vi "Autonomous State Machine .vi"   [LabVIEW 2014]
doc: "This VI is called when autonomous begins, and will automatically be terminated when autonomous ends. You can carry out timed or sensor driven robot movement independently without needing to return to the caller."
uses:
  <vilib>/Rock Robotics/WPI/RobotDrive/WPI_RobotDriveGetSetRefNum.vi
  Robot Global Data.vi
panel:
  # "Be sure to right-click and choose Data Operations>>Make Current Value default if you want to save the array values with the VI"
types:
  T1 = typedef "WPI_MotorControlDeviceRef.ctl" = cluster{"DeviceStatus":errorcluster, "Type":T2, "PWM":cluster{"Controller":T3, "PWM Channel":T4, "DeadBand":T5}, "CAN":cluster{"Device Number":u8, "Control Mode":T6, "Semaphore":T7, "Max Vout":dbl, "TalonSRX Control Mode":T8}, "Invert":bool, "TransformRef":T9, "InvTransformRef":T9}
  T2 = typedef "WPI_MotorControlType.ctl" = enum16{"PWM", "CAN", "CANTalonSRX"}
  T3 = typedef "FPGA_TypedefDigitalModule.ctl" = enum16{"Controller 1"}
  T4 = typedef "FPGA_DIOPWMChannel.ctl" = enum8{"PWM 0", "PWM 1", "PWM 2", "PWM 3", "PWM 4", "PWM 5", "PWM 6", "PWM 7", "PWM 8", "PWM 9", "PWM MXP 0", "PWM MXP 1", "PWM MXP 2", "PWM MXP 3", "PWM MXP 4", "PWM MXP 5", "PWM MXP 6", "PWM MXP 7", "PWM MXP 8", "PWM MXP 9", "Invalid"}
  T5 = typedef "WPI_PWMDeadband.ctl" = cluster{"Name":string, "maxPositivePwm":i32, "minPositivePwm":i32, "centerPwm":i32, "maxNegativePwm":i32, "minNegativePwm":i32, "angularRange":u16}
  T6 = typedef "WPI_CANJaguar_ControlMode.ctl" = enum8{"Percent VBus", "Current", "Speed", "Position", "Voltage"}
  T7 = typedef "Semaphore RefNum" = refnum<k1>
  T8 = typedef "WPI_CANTalonSRX_APIControlMode.ctl" = enum8{"Percent VBus", "Speed", "Position", "Slave", "Unchanged / Invalid"}
  T9 = typedef "WPI_PWMTransform_ConPane.ctl" = refnum<vi>
  T10 = typedef "WPI_RobotDriveDevRef.ctl" = cluster{"DevStatus":errorcluster, "Motors[]":T1[], "Square Inputs":bool, "Max Output":dbl}
  T11 = typedef "WPI_DigitalInputDevRef.ctl" = cluster{"DevStatus":errorcluster, "DIO Channel":T12, "Controller":T3}
  T12 = typedef "FPGA_DIOChannel.ctl" = enum8{"DIO 0", "DIO 1", "DIO 2", "DIO 3", "DIO 4", "DIO 5", "DIO 6", "DIO 7", "DIO 8", "DIO 9", "DIO MXP 0", "DIO MXP 1", "DIO MXP 2", "DIO MXP 3", "DIO MXP 4", "DIO MXP 5", "DIO MXP 6", "DIO MXP 7", "DIO MXP 8", "DIO MXP 9", "DIO MXP 10", "DIO MXP 11", "DIO MXP 12", "DIO MXP 13", "DIO MXP 14", "DIO MXP 15", "Invalid"}
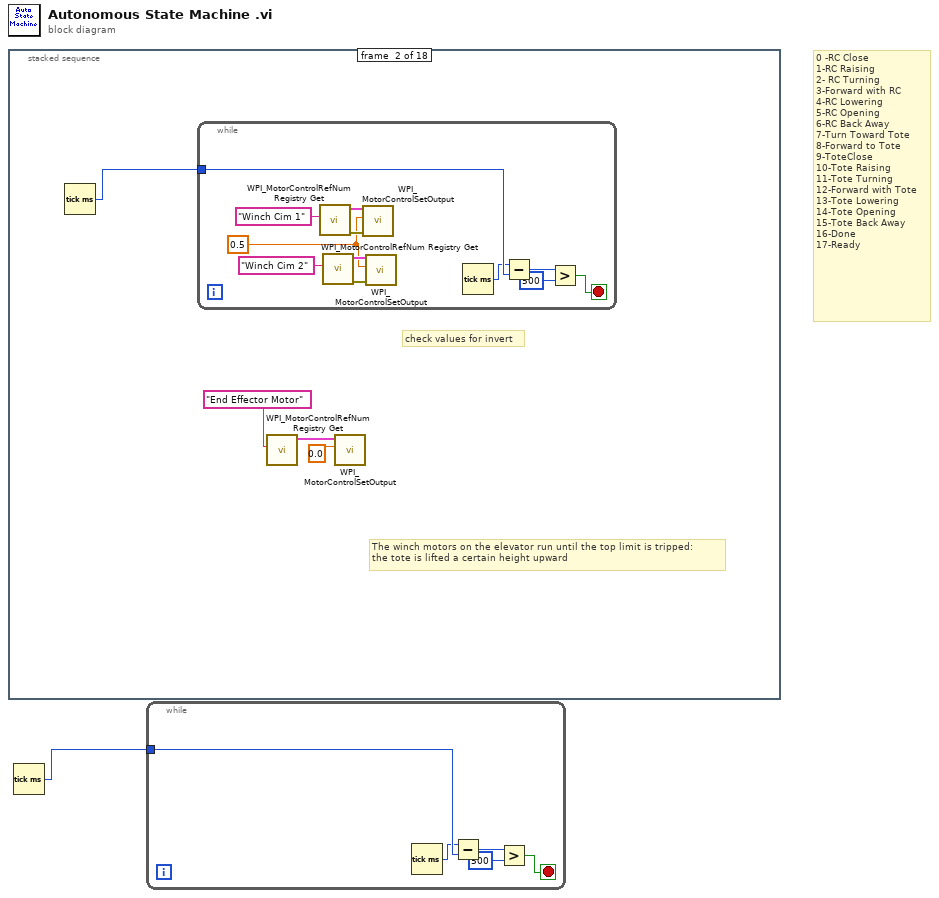
[diagram p0: block diagram]
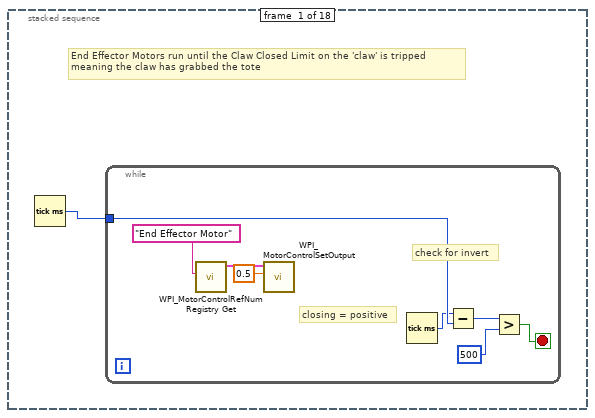
[diagram p2: hidden frame]
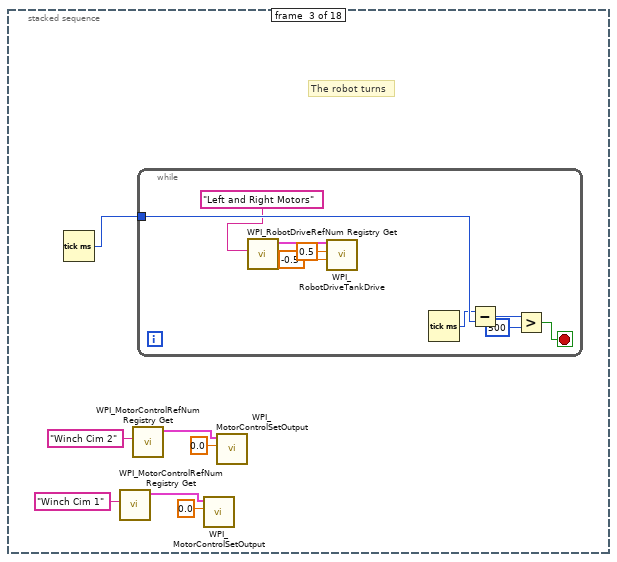
[diagram p3: hidden frame]
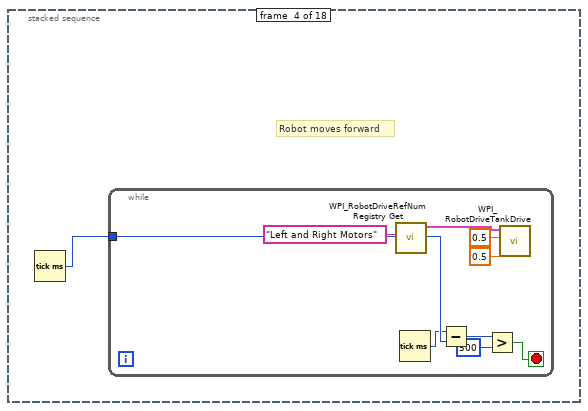
[diagram p4: hidden frame]
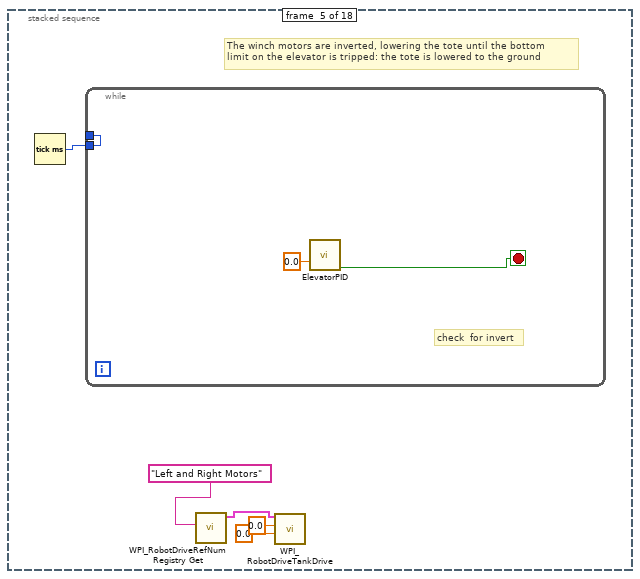
[diagram p5: hidden frame]
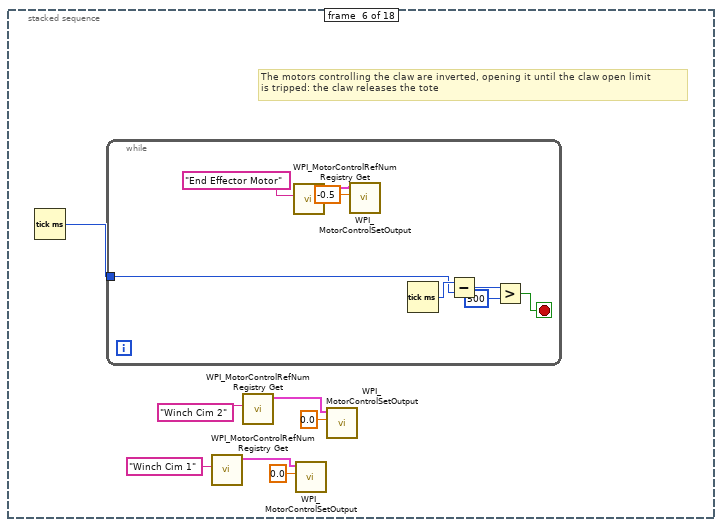
[diagram p6: hidden frame]
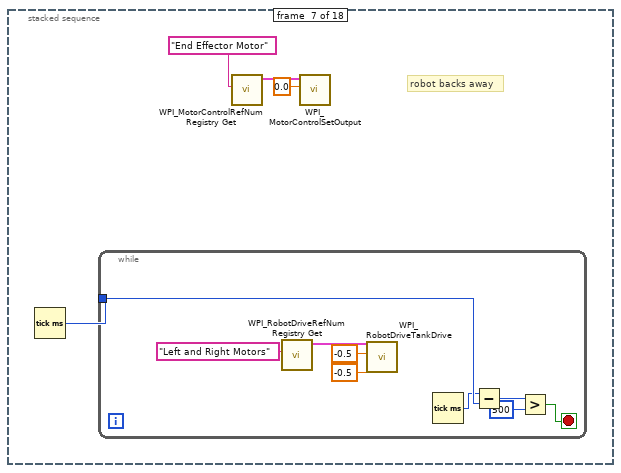
[diagram p7: hidden frame]
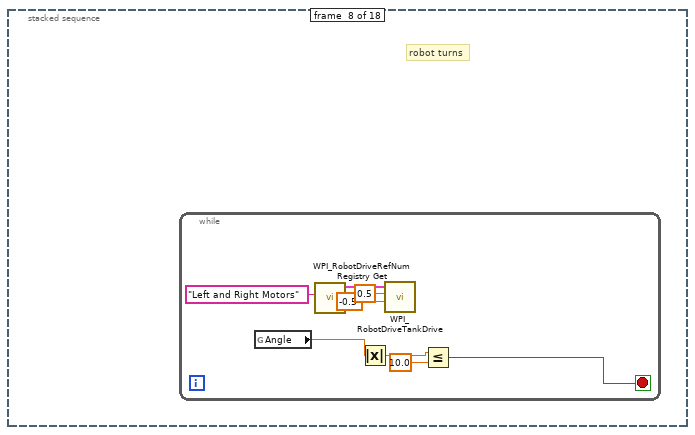
[diagram p8: hidden frame]
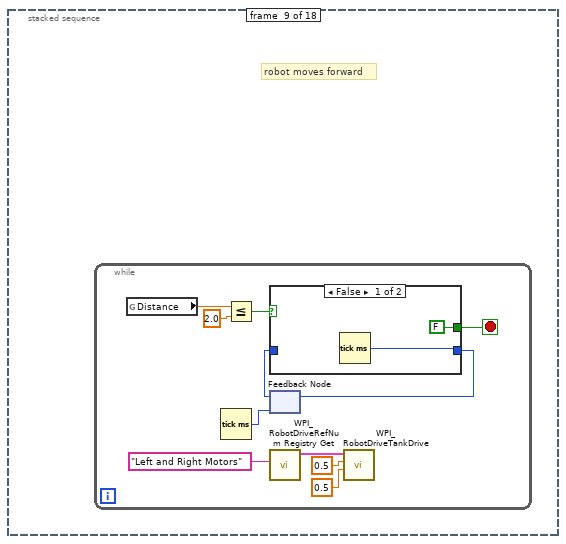
[diagram p9: hidden frame]
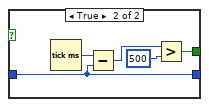
[diagram p10: hidden frame]
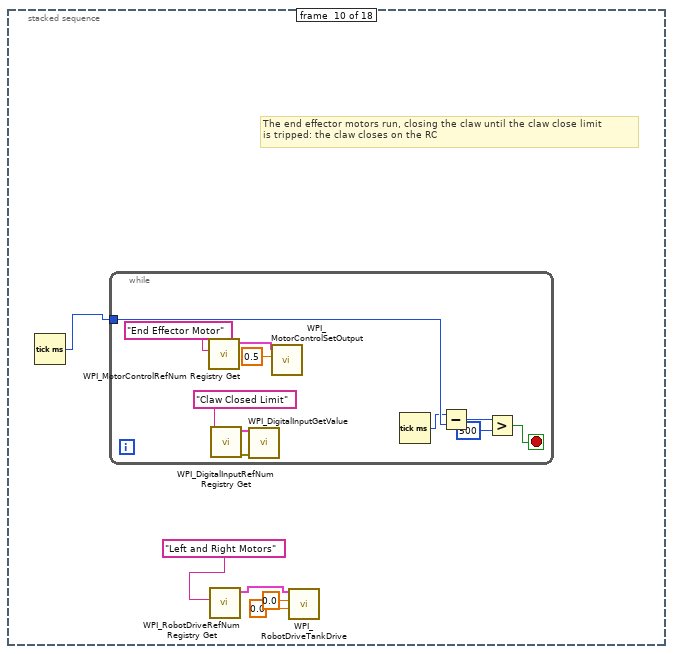
[diagram p11: hidden frame]
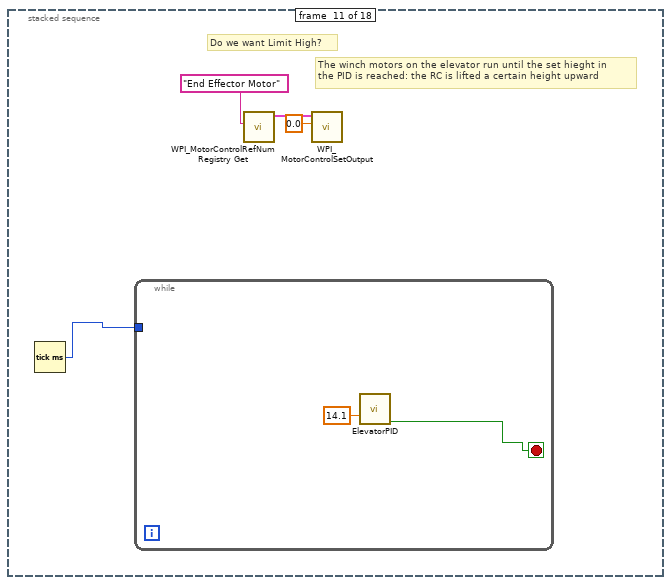
[diagram p12: hidden frame]
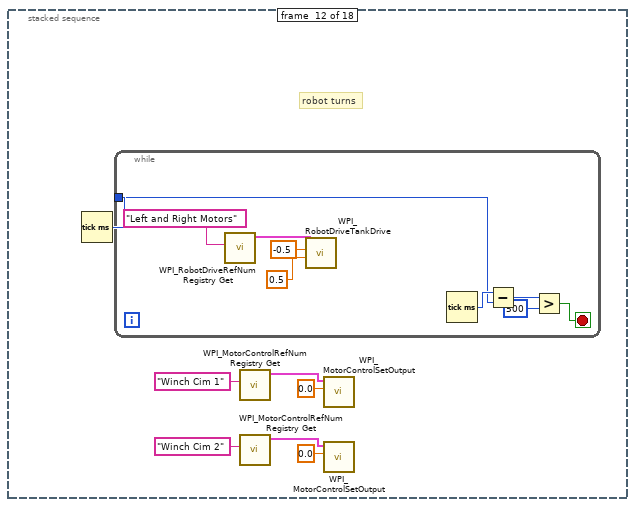
[diagram p13: hidden frame]
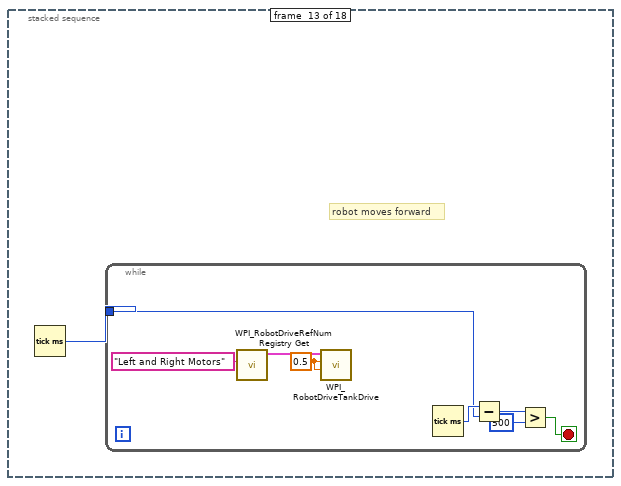
[diagram p14: hidden frame]
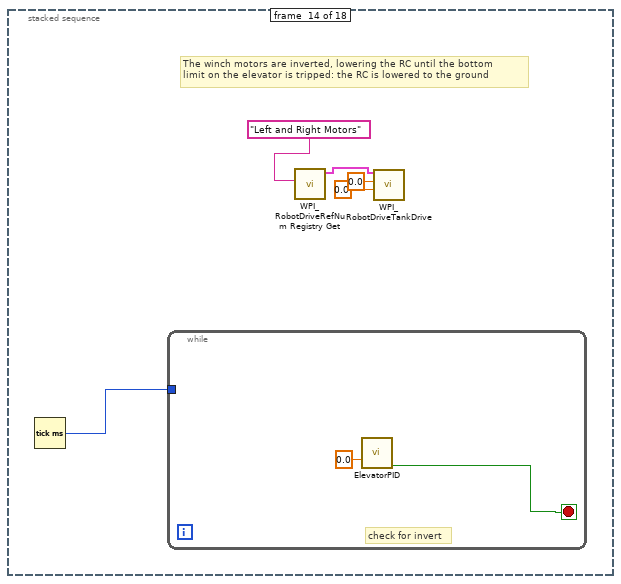
[diagram p15: hidden frame]
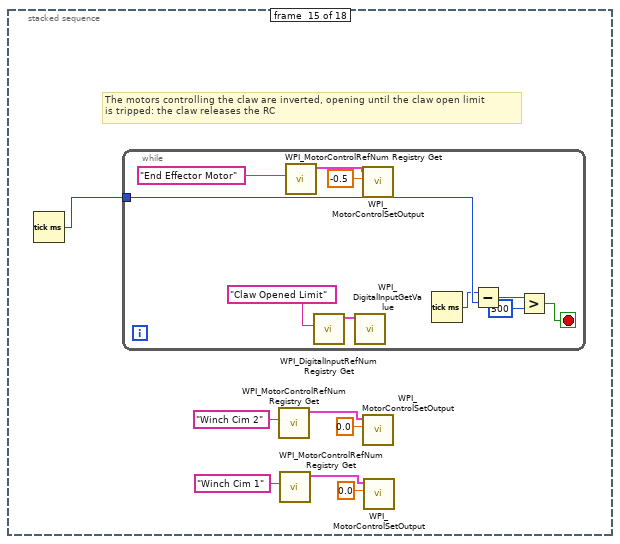
[diagram p16: hidden frame]
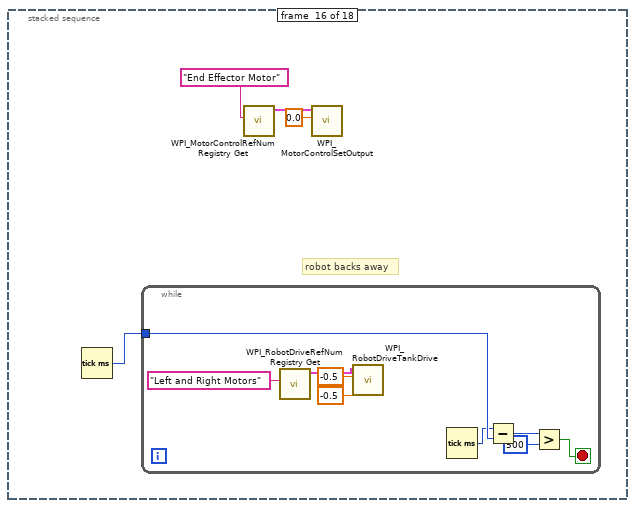
[diagram p17: hidden frame]
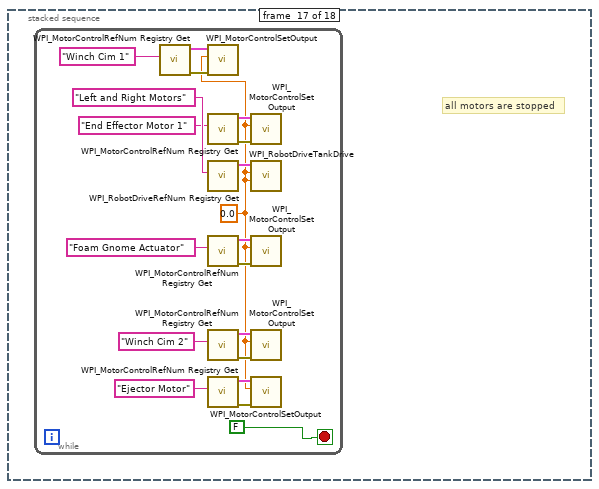
[diagram p18: hidden frame]
diagram:
  # "0 -RC Close\n1-RC Raising\n2- RC Turning\n3-Forward with RC\n4-RC Lowering\n5-RC Opening\n6-RC Back Away\n7-Turn Toward Tote\n8-Forward to Tote\n9-ToteClose\n10-Tote Raising\n11-Tote Turning\n12-Forward with Tote\n13-Tote Lowering\n14-Tote Opening\n15-Tote Back Away\n16-Done\n17-Ready"
  n1 = stacked-sequence {
    frame #0 {
      # "End Effector Motors run until the Claw Closed Limit on the 'claw' is tripped\nmeaning the claw has grabbed the tote"
      n2 = Tick Count (ms)() -> (millisecond timer value=w2:u32)
      n3 = while {
        tunnel: w2 -> [w7]
        stop <- w8 stop-if-true
        # "closing = positive"
        # "check for invert"
        n4 = call <vilib>:"WPI_MotorControlRefNum Registry Get.vi"("refnum name"="End Effector Motor") -> ("MotorControlDevRef"=w3:T1)  [unwired: 9 in, 1 out]
        n5 = call <vilib>:"WPI_MotorControlSetOutput.vi"("Output"=0.5, "MotorControlDevRef"=w3) -> ()  [unwired: 7 in, 3 out]
        n6 = Tick Count (ms)() -> (millisecond timer value=w6:u32)
        n7 = Subtract(x=w6, y=w7) -> (x-y=w10:u32)
        n8 = Greater?(x=w10, y=u32 500) -> (0:w8:bool)
      }
    }
    frame #1 {
      # "The winch motors on the elevator run until the top limit is tripped: \nthe tote is lifted a certain height upward"
      # "check values for invert"
      n9 = Tick Count (ms)() -> (millisecond timer value=w11:u32)
      n10 = while {
        tunnel: w11 -> [w23]
        stop <- w24 stop-if-true
        w15 = 0.5
        n11 = call <vilib>:"WPI_MotorControlRefNum Registry Get.vi"("refnum name"="Winch Cim 1") -> ("error out"=w20:errorcluster, "MotorControlDevRef"=w19:T1)  [unwired: 9 in]
        n12 = call <vilib>:"WPI_MotorControlRefNum Registry Get.vi"("refnum name"="Winch Cim 2") -> ("error out"=w17:errorcluster, "MotorControlDevRef"=w16:T1)  [unwired: 9 in]
        n13 = call <vilib>:"WPI_MotorControlSetOutput.vi"("error in (no error)"=w20, "Output"=w15, "MotorControlDevRef"=w19) -> ()  [unwired: 6 in, 3 out]
        n14 = call <vilib>:"WPI_MotorControlSetOutput.vi"("error in (no error)"=w17, "Output"=w15, "MotorControlDevRef"=w16) -> ()  [unwired: 6 in, 3 out]
        n15 = Tick Count (ms)() -> (millisecond timer value=w22:u32)
        n16 = Subtract(x=w22, y=w23) -> (x-y=w26:u32)
        n17 = Greater?(x=w26, y=u32 500) -> (0:w24:bool)
      }
      n18 = call <vilib>:"WPI_MotorControlRefNum Registry Get.vi"("refnum name"="End Effector Motor") -> ("MotorControlDevRef"=w12:T1)  [unwired: 9 in, 1 out]
      n19 = call <vilib>:"WPI_MotorControlSetOutput.vi"("Output"=0.0, "MotorControlDevRef"=w12) -> ()  [unwired: 7 in, 3 out]
    }
    frame #2 {
      # "The robot turns"
      n20 = Tick Count (ms)() -> (millisecond timer value=w33:u32)
      n21 = call <vilib>:"WPI_MotorControlRefNum Registry Get.vi"("refnum name"="Winch Cim 1") -> ("MotorControlDevRef"=w28:T1)  [unwired: 9 in, 1 out]
      n22 = call <vilib>:"WPI_MotorControlRefNum Registry Get.vi"("refnum name"="Winch Cim 2") -> ("MotorControlDevRef"=w31:T1)  [unwired: 9 in, 1 out]
      n23 = while {
        tunnel: w33 -> [w39]
        stop <- w40 stop-if-true
        n24 = call <vilib>:"WPI_RobotDriveRefNum Registry Get.vi"("refnum name"="Left and Right Motors") -> ("RobotDriveDevRef"=w37:T10)  [unwired: 9 in, 1 out]
        n25 = call <vilib>:"WPI_RobotDriveTankDrive.vi"("Right axis value"=-0.5, "Left axis value"=0.5, "RobotDriveDevRef"=w37) -> ()  [unwired: 6 in, 3 out]
        n26 = Tick Count (ms)() -> (millisecond timer value=w38:u32)
        n27 = Subtract(x=w38, y=w39) -> (x-y=w42:u32)
        n28 = Greater?(x=w42, y=u32 500) -> (0:w40:bool)
      }
      n29 = call <vilib>:"WPI_MotorControlSetOutput.vi"("Output"=0.0, "MotorControlDevRef"=w28) -> ()  [unwired: 7 in, 3 out]
      n30 = call <vilib>:"WPI_MotorControlSetOutput.vi"("Output"=0.0, "MotorControlDevRef"=w31) -> ()  [unwired: 7 in, 3 out]
    }
    frame #3 {
      # "Robot moves forward"
      n31 = Tick Count (ms)() -> (millisecond timer value=w43:u32)
      n32 = while {
        tunnel: w43 -> [w49]
        stop <- w50 stop-if-true
        n33 = call <vilib>:"WPI_RobotDriveRefNum Registry Get.vi"("refnum name"="Left and Right Motors") -> ("RobotDriveDevRef"=w47:T10)  [unwired: 9 in, 1 out]
        n34 = Tick Count (ms)() -> (millisecond timer value=w48:u32)
        n35 = Subtract(x=w48, y=w49) -> (x-y=w52:u32)
        n36 = Greater?(x=w52, y=u32 500) -> (0:w50:bool)
        n37 = call <vilib>:"WPI_RobotDriveTankDrive.vi"("Right axis value"=0.5, "Left axis value"=0.5, "RobotDriveDevRef"=w47) -> ()  [unwired: 6 in, 3 out]
      }
    }
    frame #4 {
      # "The winch motors are inverted, lowering the tote until the bottom \nlimit on the elevator is tripped: the tote is lowered to the ground"
      n38 = Tick Count (ms)() -> (millisecond timer value=w57:u32)
      n39 = while {
        tunnel: [w60] -> _
        tunnel: w57 -> [w60]
        stop <- w58 stop-if-true
        # "check  for invert"
        n40 = call "ElevatorPID.vi"("Elevator Setpoint"=0.0) -> ("At Setpoint"=w58:bool)  [unwired: 14 in]
      }
      n41 = call <vilib>:"WPI_RobotDriveRefNum Registry Get.vi"("refnum name"="Left and Right Motors") -> ("RobotDriveDevRef"=w56:T10)  [unwired: 9 in, 1 out]
      n42 = call <vilib>:"WPI_RobotDriveTankDrive.vi"("Right axis value"=0.0, "Left axis value"=0.0, "RobotDriveDevRef"=w56) -> ()  [unwired: 6 in, 3 out]
    }
    frame #5 {
      # "The motors controlling the claw are inverted, opening it until the claw open limit\nis tripped: the claw releases the tote"
      n43 = Tick Count (ms)() -> (millisecond timer value=w67:u32)
      n44 = while {
        tunnel: w67 -> [w68]
        stop <- w73 stop-if-true
        n45 = call <vilib>:"WPI_MotorControlRefNum Registry Get.vi"("refnum name"="End Effector Motor") -> ("MotorControlDevRef"=w70:T1)  [unwired: 9 in, 1 out]
        n46 = call <vilib>:"WPI_MotorControlSetOutput.vi"("Output"=-0.5, "MotorControlDevRef"=w70) -> ()  [unwired: 7 in, 3 out]
        n47 = Tick Count (ms)() -> (millisecond timer value=w72:u32)
        n48 = Subtract(x=w72, y=w68) -> (x-y=w75:u32)
        n49 = Greater?(x=w75, y=u32 500) -> (0:w73:bool)
      }
      n50 = call <vilib>:"WPI_MotorControlRefNum Registry Get.vi"("refnum name"="Winch Cim 1") -> ("MotorControlDevRef"=w62:T1)  [unwired: 9 in, 1 out]
      n51 = call <vilib>:"WPI_MotorControlRefNum Registry Get.vi"("refnum name"="Winch Cim 2") -> ("MotorControlDevRef"=w65:T1)  [unwired: 9 in, 1 out]
      n52 = call <vilib>:"WPI_MotorControlSetOutput.vi"("Output"=0.0, "MotorControlDevRef"=w62) -> ()  [unwired: 7 in, 3 out]
      n53 = call <vilib>:"WPI_MotorControlSetOutput.vi"("Output"=0.0, "MotorControlDevRef"=w65) -> ()  [unwired: 7 in, 3 out]
    }
    frame #6 {
      # "robot backs away"
      n54 = Tick Count (ms)() -> (millisecond timer value=w79:u32)
      n55 = while {
        tunnel: w79 -> [w85]
        stop <- w86 stop-if-true
        n56 = call <vilib>:"WPI_RobotDriveRefNum Registry Get.vi"("refnum name"="Left and Right Motors") -> ("RobotDriveDevRef"=w83:T10)  [unwired: 9 in, 1 out]
        n57 = call <vilib>:"WPI_RobotDriveTankDrive.vi"("Right axis value"=-0.5, "Left axis value"=-0.5, "RobotDriveDevRef"=w83) -> ()  [unwired: 6 in, 3 out]
        n58 = Tick Count (ms)() -> (millisecond timer value=w84:u32)
        n59 = Subtract(x=w84, y=w85) -> (x-y=w88:u32)
        n60 = Greater?(x=w88, y=u32 500) -> (0:w86:bool)
      }
      n61 = call <vilib>:"WPI_MotorControlRefNum Registry Get.vi"("refnum name"="End Effector Motor") -> ("MotorControlDevRef"=w76:T1)  [unwired: 9 in, 1 out]
      n62 = call <vilib>:"WPI_MotorControlSetOutput.vi"("Output"=0.0, "MotorControlDevRef"=w76) -> ()  [unwired: 7 in, 3 out]
    }
    frame #7 {
      # "robot turns"
      n63 = while {
        stop <- w89 stop-if-true
        n64 = global read "Robot Global Data.vi" "Angle"() -> (w90:dbl)
        n65 = call <vilib>:"WPI_RobotDriveRefNum Registry Get.vi"("refnum name"="Left and Right Motors") -> ("RobotDriveDevRef"=w96:T10)  [unwired: 9 in, 1 out]
        n66 = Absolute Value(x=w90) -> (abs(x)=w91:dbl)
        n67 = call <vilib>:"WPI_RobotDriveTankDrive.vi"("Right axis value"=-0.5, "Left axis value"=0.5, "RobotDriveDevRef"=w96) -> ()  [unwired: 6 in, 3 out]
        n68 = Less Or Equal?(x=w91, y=10.0) -> (x <= y?=w89:bool)
      }
    }
    frame #8 {
      # "robot moves forward"
      n69 = while {
        stop <- w100 stop-if-true
        n70 = global read "Robot Global Data.vi" "Distance"() -> (w103:dbl)
        n71 = Tick Count (ms)() -> (millisecond timer value=w97:u32)
        n72 = Less Or Equal?(x=w103, y=2.0) -> (x <= y?=w101:bool)
        n73 = feedback #1(w97) -> (w98:u32)
        n74 = case shown="False" w101 {
          tunnel: [w108 w110] -> w99
          tunnel: [FALSE w111] -> w100
          tunnel: w98 -> [_ w110]
          frame False {
            n75 = Tick Count (ms)() -> (millisecond timer value=w108:u32)
          }
          frame True {
            n76 = Tick Count (ms)() -> (millisecond timer value=w112:u32)
            n77 = Subtract(x=w112, y=w110) -> (x-y=w114:u32)
            n78 = Greater?(x=w114, y=u32 500) -> (0:w111:bool)
          }
        }
        n79 = feedback-in #1(w99) -> ()
        n80 = call <vilib>:"WPI_RobotDriveRefNum Registry Get.vi"("refnum name"="Left and Right Motors") -> ("RobotDriveDevRef"=w107:T10)  [unwired: 9 in, 1 out]
        n81 = call <vilib>:"WPI_RobotDriveTankDrive.vi"("Right axis value"=0.5, "Left axis value"=0.5, "RobotDriveDevRef"=w107) -> ()  [unwired: 6 in, 3 out]
      }
    }
    frame #9 {
      # "The end effector motors run, closing the claw until the claw close limit \nis tripped: the claw closes on the RC"
      n82 = Tick Count (ms)() -> (millisecond timer value=w119:u32)
      n83 = while {
        tunnel: w119 -> [w127]
        stop <- w128 stop-if-true
        n84 = call <vilib>:"WPI_MotorControlRefNum Registry Get.vi"("refnum name"="End Effector Motor") -> ("MotorControlDevRef"=w123:T1)  [unwired: 9 in, 1 out]
        n85 = call <vilib>:"WPI_DigitalInputRefNum Registry Get.vi"("refnum name"="Claw Closed Limit") -> ("error out"=w121:errorcluster, "DigitalInputDevRef"=w122:T11)  [unwired: 9 in]
        n86 = call <vilib>:"WPI_DigitalInputGetValue.vi"("error in (no error)"=w121, "DigitalInputDevRef"=w122) -> ()  [unwired: 7 in, 3 out]
        n87 = call <vilib>:"WPI_MotorControlSetOutput.vi"("Output"=0.5, "MotorControlDevRef"=w123) -> ()  [unwired: 7 in, 3 out]
        n88 = Tick Count (ms)() -> (millisecond timer value=w126:u32)
        n89 = Subtract(x=w126, y=w127) -> (x-y=w130:u32)
        n90 = Greater?(x=w130, y=u32 500) -> (0:w128:bool)
      }
      n91 = call <vilib>:"WPI_RobotDriveRefNum Registry Get.vi"("refnum name"="Left and Right Motors") -> ("RobotDriveDevRef"=w118:T10)  [unwired: 9 in, 1 out]
      n92 = call <vilib>:"WPI_RobotDriveTankDrive.vi"("Right axis value"=0.0, "Left axis value"=0.0, "RobotDriveDevRef"=w118) -> ()  [unwired: 6 in, 3 out]
    }
    frame #10 {
      # "The winch motors on the elevator run until the set hieght in \nthe PID is reached: the RC is lifted a certain height upward"
      # "Do we want Limit High?"
      n93 = Tick Count (ms)() -> (millisecond timer value=w134:u32)
      n94 = while {
        tunnel: w134 -> [_]
        stop <- w135 stop-if-true
        n95 = call "ElevatorPID.vi"("Elevator Setpoint"=14.1) -> ("At Setpoint"=w135:bool)  [unwired: 14 in]
      }
      n96 = call <vilib>:"WPI_MotorControlRefNum Registry Get.vi"("refnum name"="End Effector Motor") -> ("MotorControlDevRef"=w133:T1)  [unwired: 9 in, 1 out]
      n97 = call <vilib>:"WPI_MotorControlSetOutput.vi"("Output"=0.0, "MotorControlDevRef"=w133) -> ()  [unwired: 7 in, 3 out]
    }
    frame #11 {
      # "robot turns"
      n98 = Tick Count (ms)() -> (millisecond timer value=w143:u32)
      n99 = while {
        tunnel: w143 -> [w148]
        stop <- w150 stop-if-true
        n100 = call <vilib>:"WPI_RobotDriveRefNum Registry Get.vi"("refnum name"="Left and Right Motors") -> ("RobotDriveDevRef"=w147:T10)  [unwired: 9 in, 1 out]
        n101 = call <vilib>:"WPI_RobotDriveTankDrive.vi"("Right axis value"=0.5, "Left axis value"=-0.5, "RobotDriveDevRef"=w147) -> ()  [unwired: 6 in, 3 out]
        n102 = Tick Count (ms)() -> (millisecond timer value=w149:u32)
        n103 = Subtract(x=w149, y=w148) -> (x-y=w152:u32)
        n104 = Greater?(x=w152, y=u32 500) -> (0:w150:bool)
      }
      n105 = call <vilib>:"WPI_MotorControlRefNum Registry Get.vi"("refnum name"="Winch Cim 1") -> ("MotorControlDevRef"=w141:T1)  [unwired: 9 in, 1 out]
      n106 = call <vilib>:"WPI_MotorControlRefNum Registry Get.vi"("refnum name"="Winch Cim 2") -> ("MotorControlDevRef"=w138:T1)  [unwired: 9 in, 1 out]
      n107 = call <vilib>:"WPI_MotorControlSetOutput.vi"("Output"=0.0, "MotorControlDevRef"=w141) -> ()  [unwired: 7 in, 3 out]
      n108 = call <vilib>:"WPI_MotorControlSetOutput.vi"("Output"=0.0, "MotorControlDevRef"=w138) -> ()  [unwired: 7 in, 3 out]
    }
    frame #12 {
      # "robot moves forward"
      n109 = Tick Count (ms)() -> (millisecond timer value=w153:u32)
      n110 = while {
        tunnel: w153 -> [w157]
        stop <- w159 stop-if-true
        w154 = 0.5 ("Left axis value")
        n111 = call <vilib>:"WPI_RobotDriveRefNum Registry Get.vi"("refnum name"="Left and Right Motors") -> ("RobotDriveDevRef"=w156:T10)  [unwired: 9 in, 1 out]
        n112 = call <vilib>:"WPI_RobotDriveTankDrive.vi"("Right axis value"=w154, "Left axis value"=w154, "RobotDriveDevRef"=w156) -> ()  [unwired: 6 in, 3 out]
        n113 = Tick Count (ms)() -> (millisecond timer value=w158:u32)
        n114 = Subtract(x=w158, y=w157) -> (x-y=w161:u32)
        n115 = Greater?(x=w161, y=u32 500) -> (0:w159:bool)
      }
    }
    frame #13 {
      # "The winch motors are inverted, lowering the RC until the bottom \nlimit on the elevator is tripped: the RC is lowered to the ground"
      n116 = Tick Count (ms)() -> (millisecond timer value=w166:u32)
      n117 = while {
        tunnel: w166 -> [_]
        stop <- w167 stop-if-true
        # "check for invert"
        n118 = call "ElevatorPID.vi"("Elevator Setpoint"=0.0) -> ("At Setpoint"=w167:bool)  [unwired: 14 in]
      }
      n119 = call <vilib>:"WPI_RobotDriveRefNum Registry Get.vi"("refnum name"="Left and Right Motors") -> ("RobotDriveDevRef"=w165:T10)  [unwired: 9 in, 1 out]
      n120 = call <vilib>:"WPI_RobotDriveTankDrive.vi"("Right axis value"=0.0, "Left axis value"=0.0, "RobotDriveDevRef"=w165) -> ()  [unwired: 6 in, 3 out]
    }
    frame #14 {
      # "The motors controlling the claw are inverted, opening until the claw open limit\nis tripped: the claw releases the RC"
      n121 = Tick Count (ms)() -> (millisecond timer value=w175:u32)
      n122 = while {
        tunnel: w175 -> [w182]
        stop <- w183 stop-if-true
        n123 = call <vilib>:"WPI_MotorControlRefNum Registry Get.vi"("refnum name"="End Effector Motor") -> ("MotorControlDevRef"=w176:T1)  [unwired: 9 in, 1 out]
        n124 = call <vilib>:"WPI_DigitalInputRefNum Registry Get.vi"("refnum name"="Claw Opened Limit") -> ("DigitalInputDevRef"=w179:T11)  [unwired: 9 in, 1 out]
        n125 = call <vilib>:"WPI_DigitalInputGetValue.vi"("DigitalInputDevRef"=w179) -> ()  [unwired: 8 in, 3 out]
        n126 = call <vilib>:"WPI_MotorControlSetOutput.vi"("Output"=-0.5, "MotorControlDevRef"=w176) -> ()  [unwired: 7 in, 3 out]
        n127 = Tick Count (ms)() -> (millisecond timer value=w181:u32)
        n128 = Subtract(x=w181, y=w182) -> (x-y=w185:u32)
        n129 = Greater?(x=w185, y=u32 500) -> (0:w183:bool)
      }
      n130 = call <vilib>:"WPI_MotorControlRefNum Registry Get.vi"("refnum name"="Winch Cim 2") -> ("MotorControlDevRef"=w173:T1)  [unwired: 9 in, 1 out]
      n131 = call <vilib>:"WPI_MotorControlRefNum Registry Get.vi"("refnum name"="Winch Cim 1") -> ("MotorControlDevRef"=w170:T1)  [unwired: 9 in, 1 out]
      n132 = call <vilib>:"WPI_MotorControlSetOutput.vi"("Output"=0.0, "MotorControlDevRef"=w173) -> ()  [unwired: 7 in, 3 out]
      n133 = call <vilib>:"WPI_MotorControlSetOutput.vi"("Output"=0.0, "MotorControlDevRef"=w170) -> ()  [unwired: 7 in, 3 out]
    }
    frame #15 {
      # "robot backs away"
      n134 = Tick Count (ms)() -> (millisecond timer value=w189:u32)
      n135 = while {
        tunnel: w189 -> [w195]
        stop <- w196 stop-if-true
        n136 = call <vilib>:"WPI_RobotDriveRefNum Registry Get.vi"("refnum name"="Left and Right Motors") -> ("RobotDriveDevRef"=w193:T10)  [unwired: 9 in, 1 out]
        n137 = call <vilib>:"WPI_RobotDriveTankDrive.vi"("Right axis value"=-0.5, "Left axis value"=-0.5, "RobotDriveDevRef"=w193) -> ()  [unwired: 6 in, 3 out]
        n138 = Tick Count (ms)() -> (millisecond timer value=w194:u32)
        n139 = Subtract(x=w194, y=w195) -> (x-y=w198:u32)
        n140 = Greater?(x=w198, y=u32 500) -> (0:w196:bool)
      }
      n141 = call <vilib>:"WPI_MotorControlRefNum Registry Get.vi"("refnum name"="End Effector Motor") -> ("MotorControlDevRef"=w186:T1)  [unwired: 9 in, 1 out]
      n142 = call <vilib>:"WPI_MotorControlSetOutput.vi"("Output"=0.0, "MotorControlDevRef"=w186) -> ()  [unwired: 7 in, 3 out]
    }
    frame #16 {
      # "all motors are stopped"
      n143 = while {
        stop <- FALSE stop-if-true
        w199 = 0.0
        n144 = call <vilib>:"WPI_MotorControlRefNum Registry Get.vi"("refnum name"="Winch Cim 1") -> ("error out"=w208:errorcluster, "MotorControlDevRef"=w207:T1)  [unwired: 9 in]
        n145 = call <vilib>:"WPI_MotorControlSetOutput.vi"("error in (no error)"=w208, "Output"=w199, "MotorControlDevRef"=w207) -> ()  [unwired: 6 in, 3 out]
        n146 = call <vilib>:"WPI_MotorControlRefNum Registry Get.vi"("refnum name"="End Effector Motor 1") -> ("error out"=w214:errorcluster, "MotorControlDevRef"=w213:T1)  [unwired: 9 in]
        n147 = call <vilib>:"WPI_RobotDriveRefNum Registry Get.vi"("refnum name"="Left and Right Motors") -> ("RobotDriveDevRef"=w216:T10)  [unwired: 9 in, 1 out]
        n148 = call <vilib>:"WPI_MotorControlRefNum Registry Get.vi"("refnum name"="Foam Gnome Actuator") -> ("error out"=w212:errorcluster, "MotorControlDevRef"=w211:T1)  [unwired: 9 in]
        n149 = call <vilib>:"WPI_MotorControlRefNum Registry Get.vi"("refnum name"="Winch Cim 2") -> ("error out"=w210:errorcluster, "MotorControlDevRef"=w209:T1)  [unwired: 9 in]
        n150 = call <vilib>:"WPI_MotorControlRefNum Registry Get.vi"("refnum name"="Ejector Motor") -> ("error out"=w204:errorcluster, "MotorControlDevRef"=w203:T1)  [unwired: 9 in]
        n151 = call <vilib>:"WPI_MotorControlSetOutput.vi"("error in (no error)"=w214, "Output"=w199, "MotorControlDevRef"=w213) -> ()  [unwired: 6 in, 3 out]
        n152 = call <vilib>:"WPI_RobotDriveTankDrive.vi"("Right axis value"=w199, "Left axis value"=w199, "RobotDriveDevRef"=w216) -> ()  [unwired: 6 in, 3 out]
        n153 = call <vilib>:"WPI_MotorControlSetOutput.vi"("error in (no error)"=w212, "Output"=w199, "MotorControlDevRef"=w211) -> ()  [unwired: 6 in, 3 out]
        n154 = call <vilib>:"WPI_MotorControlSetOutput.vi"("error in (no error)"=w210, "Output"=w199, "MotorControlDevRef"=w209) -> ()  [unwired: 6 in, 3 out]
        n155 = call <vilib>:"WPI_MotorControlSetOutput.vi"("error in (no error)"=w204, "Output"=w199, "MotorControlDevRef"=w203) -> ()  [unwired: 6 in, 3 out]
      }
    }
    frame #17 {
      # "absolutely nothing happens here"
    }
  }
  n156 = Tick Count (ms)() -> (millisecond timer value=w1:u32)
  n157 = while {
    tunnel: w1 -> [w219]
    stop <- w220 stop-if-true
    n158 = Tick Count (ms)() -> (millisecond timer value=w218:u32)
    n159 = Subtract(x=w218, y=w219) -> (x-y=w222:u32)
    n160 = Greater?(x=w222, y=u32 500) -> (0:w220:bool)
  }
